vi "Update Trace Tree.vi"(7 "References":T1, 8 "error in":errorcluster, 10 "Headers":string[](array[string]), 11 "Data IN":string[][](array[string])) -> (0 "error out":errorcluster, 2 "Signals":string[][](table))   [LabVIEW 2025, in "CAN-LIN Raw Bus Capture UI.lvlib"]
doc: "This VI processes the DATA and populates the Frame TREE and the Signal TABLE."
uses:
  CAN-LIN Raw Bus Capture UI.lvlib
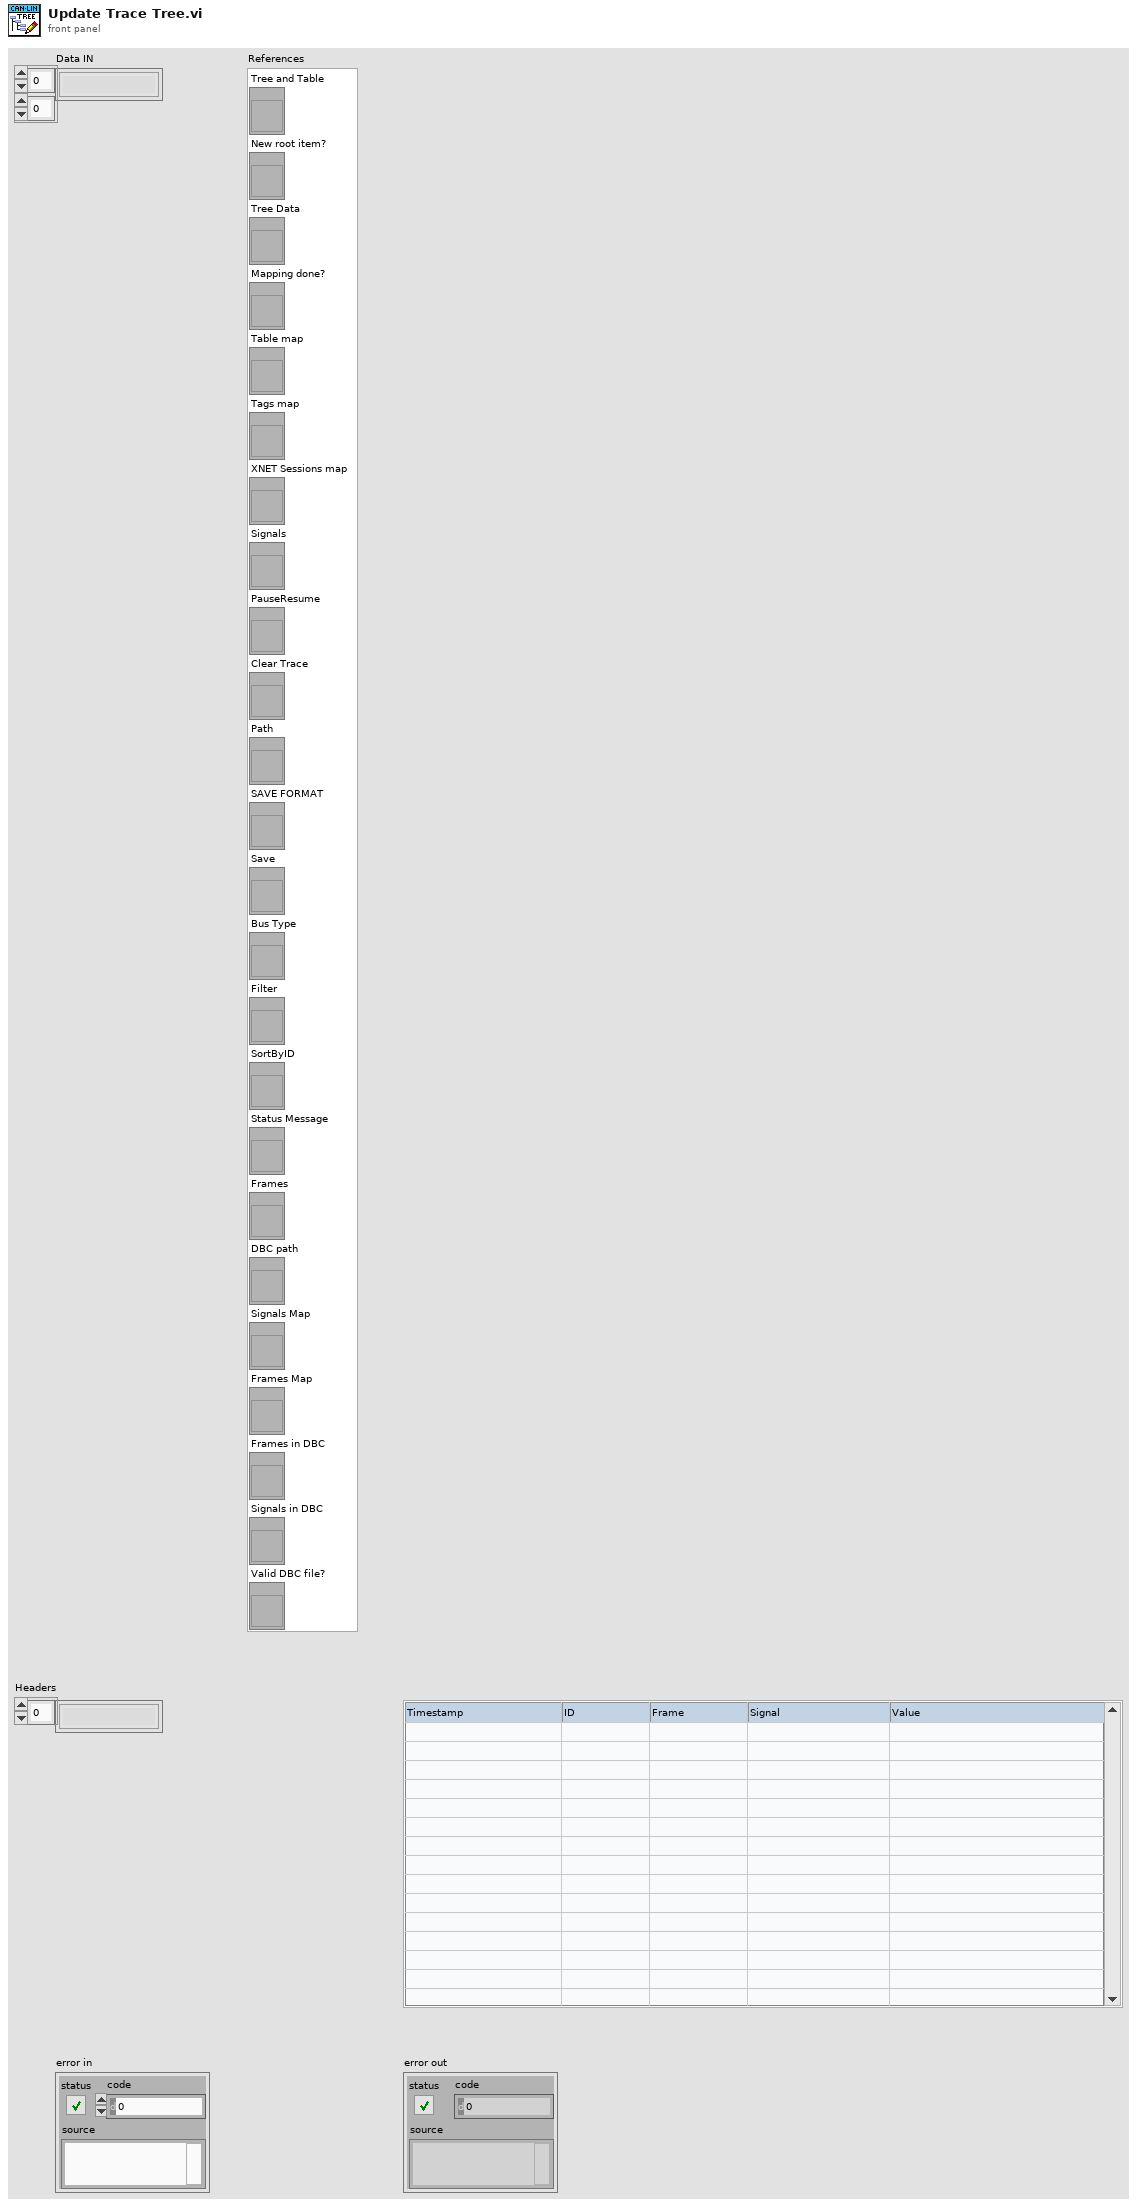
[diagram p1: front panel]
types:
  T1 = cluster{"Tree and Table":refnum<vi>, "New root item?":refnum<vi>, "Tree Data":refnum<vi>, "Mapping done?":refnum<vi>, "Table map":refnum<vi>, "Tags map":refnum<vi>, "XNET Sessions map":refnum<vi>, "Signals":refnum<vi>, "PauseResume":refnum<vi>, "Clear Trace":refnum<vi>, "Path":refnum<vi>, "SAVE FORMAT":refnum<vi>, "Save":refnum<vi>, "Bus Type":refnum<vi>, "Filter":refnum<vi>, "SortByID":refnum<vi>, "Status Message":refnum<vi>, "Frames":refnum<vi>, "DBC path":refnum<vi>, "Signals Map":refnum<vi>, "Frames Map":refnum<vi>, "Frames in DBC":refnum<vi>, "Signals in DBC":refnum<vi>, "Valid DBC file?":refnum<vi>}
  T2 = typedef "XNET Frame CAN.ctl" = cluster{"timestamp":timestamp, "payload":u8[], "identifier":u32, "type":T3, "extended?":bool, "echo?":bool}
  T3 = typedef "XNET Frame Type CAN.ctl" = u8
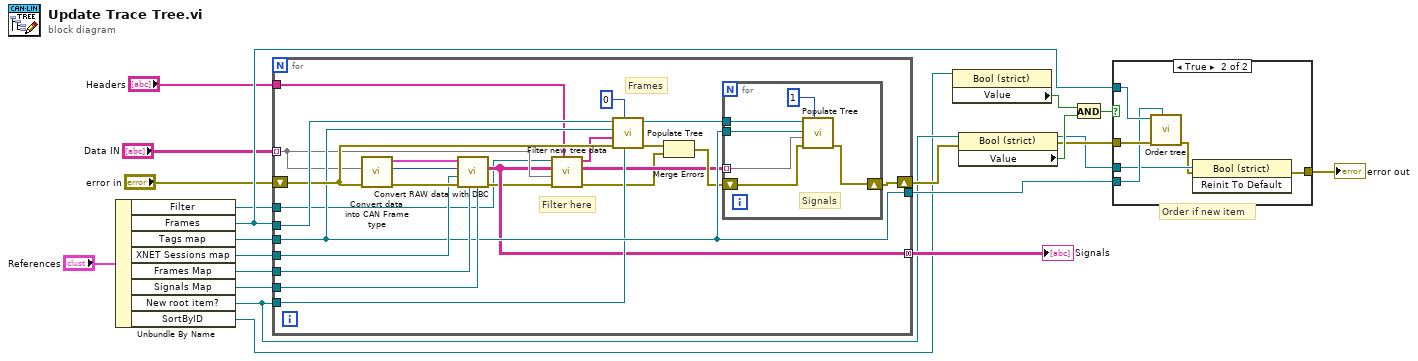
[diagram p0: block diagram]
diagram:
  # "Order if new item"
  n1 = Unbundle By Name("References") -> ("Filter"=w1:refnum<vi>, "Frames"=w12:refnum<vi>, "Tags map"=w17:refnum<vi>, "XNET Sessions map"=w19:refnum<vi>, "Frames Map"=w18:refnum<vi>, "Signals Map"=w20:refnum<vi>, "New root item?"=w8:refnum<vi>, "SortByID"=w7:refnum<vi>)
  n2 = for {
    tunnel: "Data IN" -> [w29] mode=indexing
    tunnel: w12 -> [w40]
    tunnel: [w26] -> w21 mode=concatenating
    shift-right: [w31] -> w16
    shift-left: "error in" -> [w39]
    tunnel: w18 -> [w42]
    tunnel: w20 -> [w41]
    tunnel: w17 -> [w34]
    tunnel: w19 -> [w36]
    tunnel: [w34] -> w11
    tunnel: w8 -> [w33]
    tunnel: "Headers" -> [w25]
    tunnel: w1 -> [w22]
    # "Filter here"
    # "Frames"
    n3 = call "Convert data into CAN Frame type.vi"("error in"=w39, "Frame"=w29) -> ("error out"=w38:errorcluster, "ID"=w43:u32, "CAN frame"=w37:T2)  [unwired: 7 in]
    n4 = call "Convert RAW data with DBC.vi"("Signals Map"=w41, "Frames Map"=w42, "error in"=w38, "XNET Sessions map"=w36, "ID"=w43, "Frame"=w37) -> ("error out"=w24:errorcluster, "Human Readable DATA"=w26:string[][])  [unwired: 4 in]
    n5 = call "Filter new tree data.vi"("Headers"=w25, "error in"=w24, "Root row"=w29, "Child rows"=w26, "Filter"=w22) -> ("error out"=w23:errorcluster, "Filtered child rows"=w27:string[][], "Filtered root row"=w28:string[])  [unwired: 4 in]
    n6 = call "Populate Tree.vi"("New root item?"=w33, "Indent level"=0 ("Numeric"), "error in"=w39, "Data in"=w28, "Tags map"=w34, "TreeControl in"=w40) -> ("error out"=w32:errorcluster)  [unwired: 5 in]
    n7 = Merge Errors(w32, w23) -> (w30:errorcluster)
    n8 = for {
      tunnel: w27 -> [w44] mode=indexing
      tunnel: w40 -> [w49]
      shift-right: [w47] -> w31
      shift-left: w30 -> [w48]
      tunnel: w34 -> [w46]
      # "Signals"
      n9 = call "Populate Tree.vi"("Indent level"=1, "error in"=w48, "Data in"=w44, "Tags map"=w46, "TreeControl in"=w49) -> ("error out"=w47:errorcluster)  [unwired: 6 in]
    }
  }
  "Signals" <- w21
  n10 = property class="Bool (strict)"(reference=w7) -> ("Value"=w9:bool)  [unwired: 1 in, 2 out]
  n11 = property class="Bool (strict)"(reference=w8, error in=w16) -> (reference out=w6:refnum<vi>, error out=w13:errorcluster, "Value"=w15:bool)
  n12 = And(x=w9, y=w15) -> (x .and. y?=w14:bool)
  n13 = case shown="True" w14 {
    tunnel: w13 -> [w50 w56]
    tunnel: w12 -> [_ w55]
    tunnel: w11 -> [_ w54]
    tunnel: [w50 w51] -> w10
    tunnel: w6 -> [_ w53]
    frame False {
    }
    frame True {
      n14 = call "Order tree.vi"("Tags map"=w54, "error in"=w56, "TreeControl in"=w55) -> ("error out"=w52:errorcluster)  [unwired: 8 in]
      n15 = invoke class="Bool (strict)" method="Reinit To Default"(reference=w53, error in=w52) -> (error out=w51:errorcluster)  [unwired: 1 in, 2 out]
    }
  }
  "error out" <- w10
